vi "run.remove_attachment.vi"(8 "error in":errorcluster, 11 "Client in":refnum<class "Client.lvclass">) -> (0 "error out":errorcluster, 3 "Client out":refnum<class "Client.lvclass">)   [LabVIEW 2020, in "Client.lvclass"]
doc: "Removes an attachment from the run without deleting the attachment itself."
uses:
  Client.lvclass
  Client.lvclass/Client.ctl
  client.lvlib
panel:
  in  "rid":string
  in  "attachment_rid":string
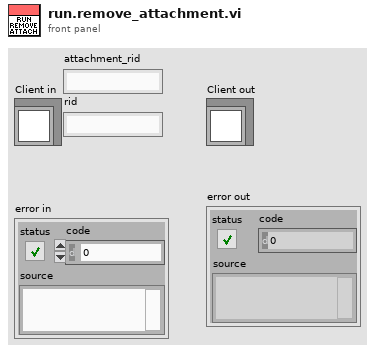
[diagram p1: front panel]
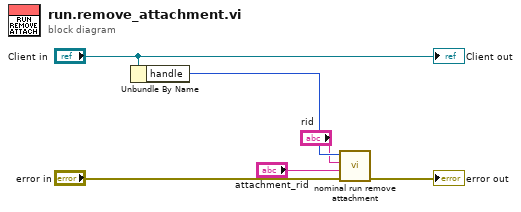
[diagram p0: block diagram]
diagram:
  n1 = Unbundle By Name("Client in") -> ("handle"=w4:i32)
  n2 = call "nominal run remove attachment.vi"("error in (no error)"="error in", "attachment_rid"="attachment_rid", "rid"="rid", "client"=w4) -> ("error out"=→"error out":errorcluster)  [unwired: 6 in, 1 out]
  "Client out" <- "Client in"
